vi "topic.set.vi"(8 "error in (no error)":errorcluster, 10 "topic":string, 11 "topic in":refnum<class "topic.lvclass">) -> (0 "error out":errorcluster, 3 "topic out":refnum<class "topic.lvclass">)   [LabVIEW 2020, in "nominal types.lvlib" / "channelFilter.lvlib" / "topic.lvclass"]
uses:
  topic.lvclass
  topic.lvclass/topic.ctl
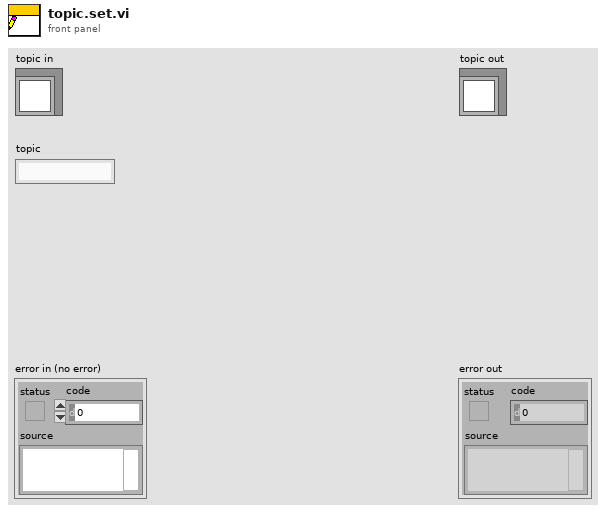
[diagram p1: front panel]
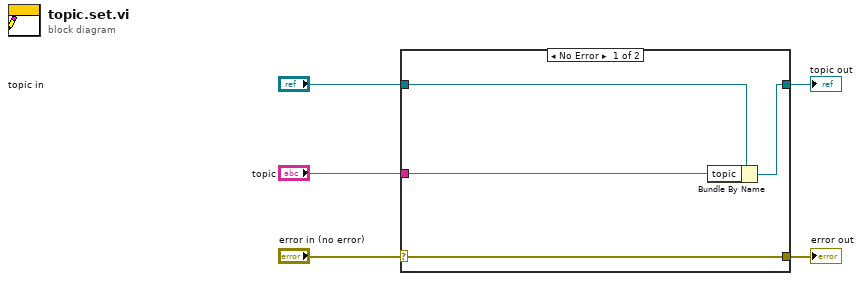
[diagram p0: block diagram]
diagram:
  n1 = case shown="No Error" "error in (no error)" {
    selector: "error in (no error)" -> [w9 w10]
    tunnel: [w9 w10] -> w4
    tunnel: [w7 w11] -> w2
    tunnel: "topic in" -> [w8 w11]
    tunnel: "topic" -> [w6 _]
    frame No Error {
      n2 = Bundle By Name(cluster=w8, "topic"=w6) -> (w7:refnum<class "topic.lvclass">)
    }
    frame Error {
    }
  }
  "error out" <- w4
  "topic out" <- w2
